vi "hw9p1_hickey.vi"() -> ()   [LabVIEW 2014]
uses:
  <vilib>/MakerHub/LINX/Private/Type Defs/User Platform.ctl
  <vilib>/MakerHub/LINX/Private/Type Defs/Interface.ctl
  <vilib>/MakerHub/LINX/Public/Peripherals/Digital/Digital Write 1 Chan.vi
  <vilib>/MakerHub/LINX/LMH-LINX.lvlib
panel:
  in  "Serial Port":refnum<visa-resource-name>="N/A"
  in  "Interface":T1
  in  "Platform":T2
  in  "stop":bool
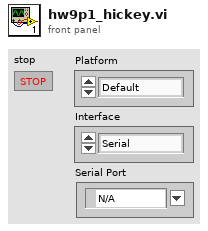
[diagram p1: front panel]
types:
  T1 = typedef "LMH-LINX.lvlib/Interface.ctl" = enum16{"Serial", "TCP"}
  T2 = typedef "LMH-LINX.lvlib/User Platform.ctl" = enum16{"Default", "LINX", "myRIO"}
  T3 = typedef "LMH-LINX.lvlib/LINX Ref.ctl" = cluster{"Platform":T4, "Interface":T1, "LINX Device Config":T5}
  T4 = typedef "LMH-LINX.lvlib/Platform.ctl" = enum16{"LINX", "myRIO"}
  T5 = typedef "LMH-LINX.lvlib/Device.lvlib/LINX Device Config.ctl" = cluster{"Interface":T1, "COM Port":refnum<visa-resource-name>, "TCP Configuration":T6, "Device Family":u8, "Device ID":u8, "Device Name":string, "TCP Ref":refnum<k5>, "Channels":T7}
  T6 = typedef "LMH-LINX.lvlib/Device.lvlib/TCP Config.ctl" = cluster{"IP Address":string, "Port":u16}
  T7 = typedef "LMH-LINX.lvlib/Channels.ctl" = cluster{"DI":u8[], "DO":u8[], "AI":u8[], "AO":u8[], "PWM":u8[], "QE":u8[], "UART":u8[], "I2C 2":u8[], "SPI":u8[], "CAN":u8[], "Servo":u8[], "AI Ref (V)":dbl, "AO Ref (V)":dbl, "AO Resolution (Bits)":u8}
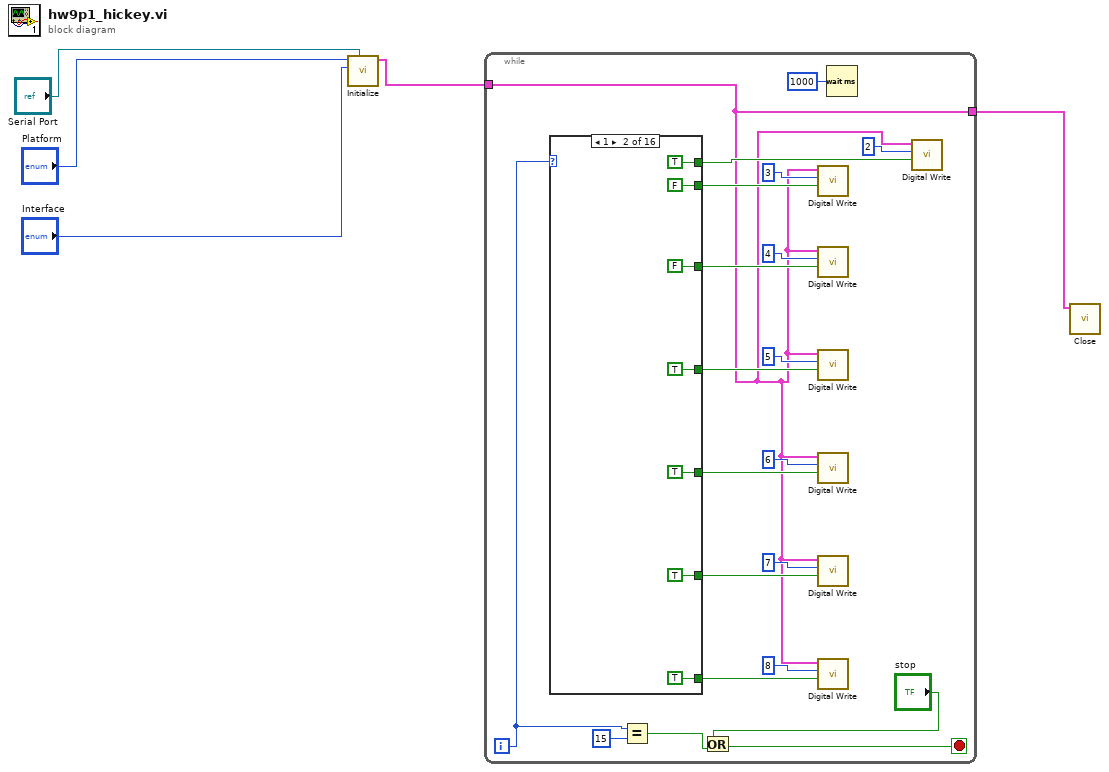
[diagram p0: block diagram]
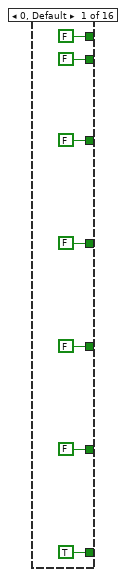
[diagram p2: hidden frame]
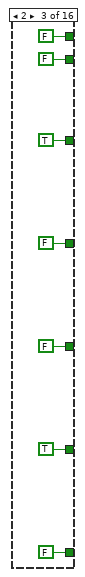
[diagram p3: hidden frame]
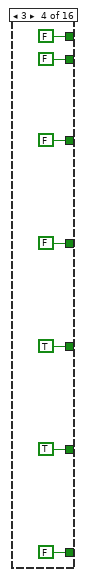
[diagram p4: hidden frame]
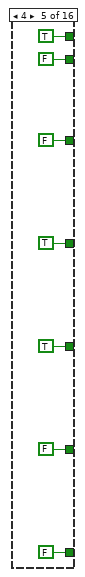
[diagram p5: hidden frame]
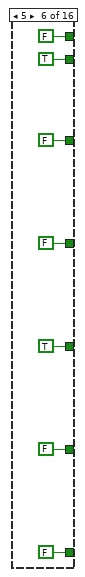
[diagram p6: hidden frame]
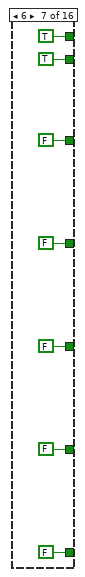
[diagram p7: hidden frame]
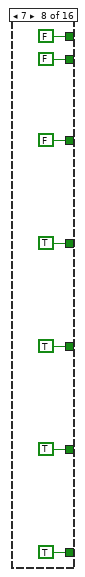
[diagram p8: hidden frame]
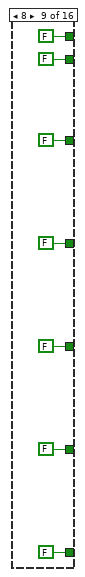
[diagram p9: hidden frame]
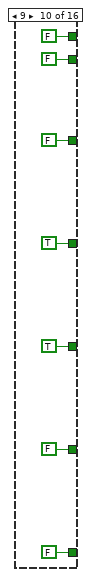
[diagram p10: hidden frame]
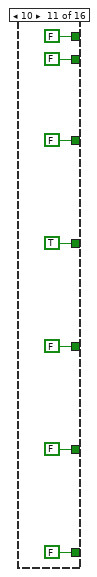
[diagram p11: hidden frame]
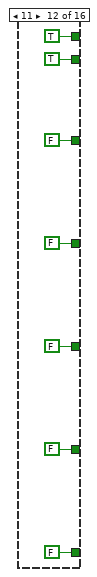
[diagram p12: hidden frame]
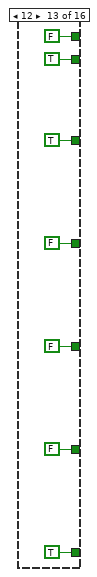
[diagram p13: hidden frame]
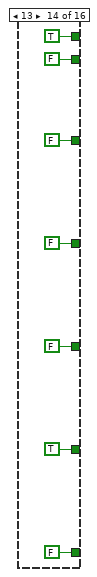
[diagram p14: hidden frame]
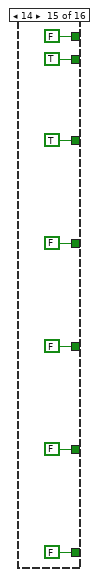
[diagram p15: hidden frame]
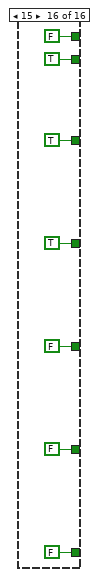
[diagram p16: hidden frame]
diagram:
  n1 = call <vilib>:"Initialize.vi"("Serial Port"="Serial Port", "Interface"="Interface", "Platform"="Platform") -> ("LINX Ref"=w4:T3)  [unwired: 6 in, 2 out]
  n2 = while {
    tunnel: [w12] -> w5
    tunnel: w4 -> [w12]
    i -> [w11]
    stop <- w7 stop-if-true
    n3 = case shown="1" w11 {
      tunnel: [FALSE FALSE FALSE FALSE FALSE TRUE TRUE FALSE FALSE FALSE FALSE TRUE TRUE FALSE TRUE TRUE] -> w13
      tunnel: [FALSE FALSE TRUE FALSE FALSE FALSE FALSE FALSE FALSE FALSE FALSE FALSE TRUE FALSE TRUE TRUE] -> w14
      tunnel: [FALSE TRUE FALSE FALSE TRUE FALSE FALSE TRUE FALSE TRUE TRUE FALSE FALSE FALSE FALSE TRUE] -> w15
      tunnel: [FALSE TRUE FALSE TRUE TRUE TRUE FALSE TRUE FALSE TRUE FALSE FALSE FALSE FALSE FALSE FALSE] -> w16
      tunnel: [FALSE TRUE TRUE TRUE FALSE FALSE FALSE TRUE FALSE FALSE FALSE FALSE FALSE TRUE FALSE FALSE] -> w17
      tunnel: [FALSE TRUE FALSE FALSE TRUE FALSE TRUE FALSE FALSE FALSE FALSE TRUE FALSE TRUE FALSE FALSE] -> w18
      tunnel: [TRUE TRUE FALSE FALSE FALSE FALSE FALSE TRUE FALSE FALSE FALSE FALSE TRUE FALSE FALSE FALSE] -> w19
      frame 0, Default {
      }
      frame 1 {
      }
      frame 2 {
      }
      frame 3 {
      }
      frame 4 {
      }
      frame 5 {
      }
      frame 6 {
      }
      frame 7 {
      }
      frame 8 {
      }
      frame 9 {
      }
      frame 10 {
      }
      frame 11 {
      }
      frame 12 {
      }
      frame 13 {
      }
      frame 14 {
      }
      frame 15 {
      }
    }
    n4 = Equal?(x=w11, y=15) -> (x = y?=w9:bool)
    n5 = Or(x="stop", y=w9) -> (x .or. y?=w7:bool)
    n6 = call-poly <vilib>:"Digital Write.vi"("Output Value"=w13, "DO Channel"=u8 3, "LINX Resource"=w12) -> ()  [unwired: 7 in, 2 out]
    n7 = call-poly <vilib>:"Digital Write.vi"("Output Value"=w14, "DO Channel"=u8 4, "LINX Resource"=w12) -> ()  [unwired: 7 in, 2 out]
    n8 = call-poly <vilib>:"Digital Write.vi"("Output Value"=w15, "DO Channel"=u8 5, "LINX Resource"=w12) -> ()  [unwired: 7 in, 2 out]
    n9 = call-poly <vilib>:"Digital Write.vi"("Output Value"=w16, "DO Channel"=u8 6, "LINX Resource"=w12) -> ()  [unwired: 7 in, 2 out]
    n10 = call-poly <vilib>:"Digital Write.vi"("Output Value"=w17, "DO Channel"=u8 7, "LINX Resource"=w12) -> ()  [unwired: 7 in, 2 out]
    n11 = call-poly <vilib>:"Digital Write.vi"("Output Value"=w19, "DO Channel"=u8 8, "LINX Resource"=w12) -> ()  [unwired: 7 in, 2 out]
    n12 = Wait (ms)(milliseconds to wait=u32 1000) -> ()  [unwired: 1 out]
    n13 = call-poly <vilib>:"Digital Write.vi"("Output Value"=w18, "DO Channel"=u8 2, "LINX Resource"=w12) -> ()  [unwired: 7 in, 2 out]
  }
  n14 = call <vilib>:"Close.vi"("LINX Resource"=w5) -> ()  [unwired: 9 in, 2 out]
